vi "Read Spreadsheet to Array.vi"() -> ()   [LabVIEW 2025]
uses:
  ca65bc03-b063-4910-9ac6-699f9501d36f.vi
  f8034dae-0d39-46bf-b97b-7079689af0b0.vi
  df198f59-68a3-411c-944b-474c12e3a6d3.vi
  <vilib>/Utility/file.llb/Read Delimited Spreadsheet (string).vi
  <vilib>/Comparison/Equal/Equal Functor/Equal Functor.lvclass
panel:
  in  "Channel":enum16{"Pressure in PSI", "Flow in LPM"}(ring)
  out "Channel Data":string[](array[string])
  in  "Specific Information":T1(ring)
  out "String from Header":string
  in  "stop":bool
  out "Test Information":string[][](array[string])
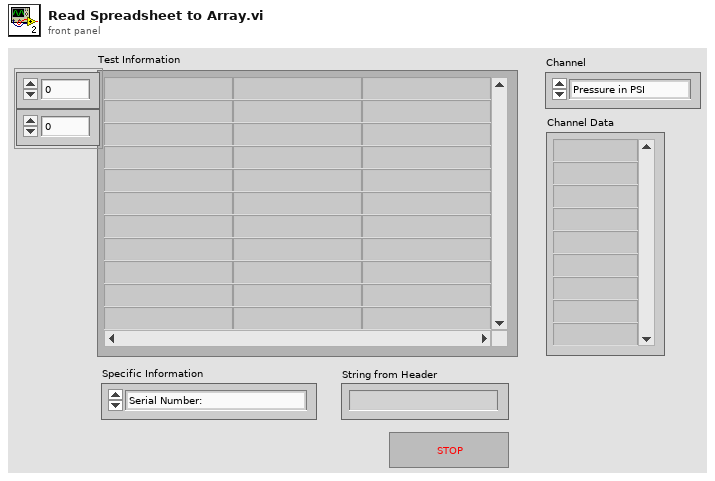
[diagram p1: front panel]
types:
  T1 = enum16{"Serial Number:", "Date:", "Test:", "Operator Name:"}
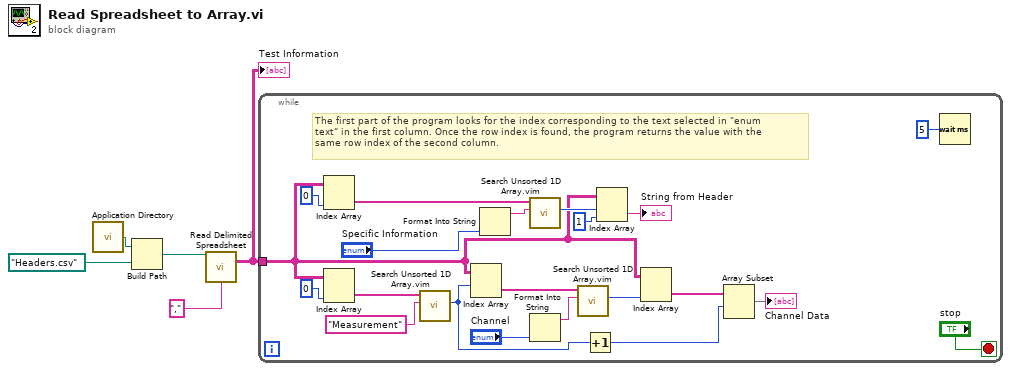
[diagram p0: block diagram]
diagram:
  n1 = call <vilib>:"Application Directory.vi"() -> ("Application Directory"=w5:path)
  n2 = Build Path(base path=w5, name or relative path=path "Headers.csv") -> (appended path=w3:path)
  n3 = call-poly <vilib>:"Read Delimited Spreadsheet.vi"("file path (dialog if empty)"=w3, "delimiter (\\t)"="," ("delimiter (\\t)")) -> ("all rows"=w1:string[][])  [unwired: 8 in, 5 out]
  "Test Information" <- w1
  n4 = while {
    tunnel: w1 -> [w11]
    stop <- "stop" stop-if-true
    # "The first part of the program looks for the index corresponding to the text selected in \"enum\ntext\" in the first column. Once the row index is found, the program returns the value with the \nsame row index of the second column."
    n5 = Index Array(array=w11, index (col)=0 ("index (row)")) -> (element=w25:string[])  [unwired: 1 in]
    n6 = Index Array(array=w11, index (col)=0 ("index (row)")) -> (element=w16:string[])  [unwired: 1 in]
    n7 = call "Search Unsorted 1D Array.vim"("element"="Measurement", "unsorted 1D array"=w16) -> ("index of element"=w7:i32)  [unwired: 9 in]
    n8 = Index Array "Index Array"(array=w11, index (row)=w7) -> (element=w12:string[])  [unwired: 1 in]
    n9 = Format Into String("Specific Information") -> (resulting string=w18:string)  [unwired: 3 in, 1 out]
    n10 = call "Search Unsorted 1D Array.vim"("element"=w18, "unsorted 1D array"=w25) -> ("index of element"=w23:i32)  [unwired: 9 in]
    n11 = Format Into String("Channel") -> (resulting string=w13:string)  [unwired: 3 in, 1 out]
    n12 = call "Search Unsorted 1D Array.vim"("element"=w13, "unsorted 1D array"=w12) -> ("index of element"=w10:i32)  [unwired: 9 in]
    n13 = Increment(x=w7) -> (x+1=w8:i32)
    n14 = Index Array(array=w11, index (row)=w23, index (col)=1) -> (element=→"String from Header":string)
    n15 = Index Array "Index Array"(array=w11, index (col)=w10) -> (element=w9:string[])  [unwired: 1 in]
    n16 = Array Subset(array=w9, index=w8) -> (→"Channel Data":string[])  [unwired: 1 in]
    n17 = Wait (ms)(milliseconds to wait=u32 5) -> ()  [unwired: 1 out]
  }
